vi "Configure Trip Line.vi"(0 "VISA resource name":refnum<visa-resource-name>, 1 "Display Position (50)":i32=50 max=100 step=1, 2 "Color":cluster{"R":i32, "G":i32, "B":i32} {"B" min=0 max=255 step=1; "G" min=0 max=255 step=1; "R" min=0 max=255 step=1}, 3 "Line Width (1: Normal)":i32(ring)=1 items=["Thin", "Normal", "Thick"], 5 "Group (1)":i32=1 min=1 max=60 step=1, 7 "Trip Line (1)":i32=1, 9 "Enable Trip Line (False)":bool, 11 "error in (no error)":errorcluster) -> (4 "VISA resource name out":refnum<visa-resource-name>, 6 "Group":i32, 8 "Trip Line":i32, 15 "error out":errorcluster)   [LabVIEW 2020, in "Yokogawa GX Series.lvlib"]
doc: "Sets the trip line for a display group.\n\nCommand: STripLine"
uses:
  <instrlib>/Yokogawa GX Series/Yokogawa GX Series.lvlib
panel:
  # "%"
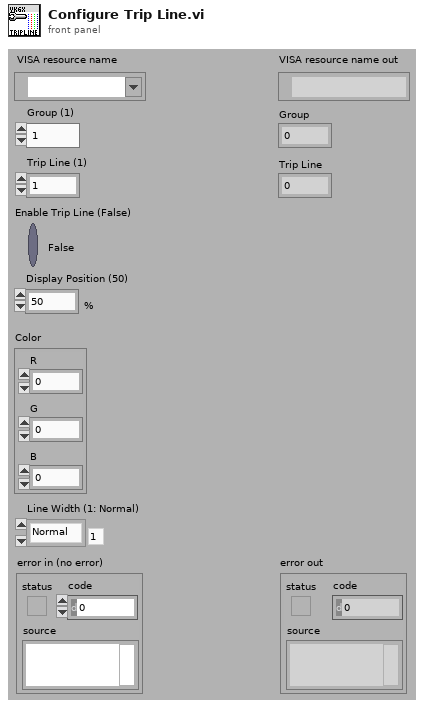
[diagram p1: front panel]
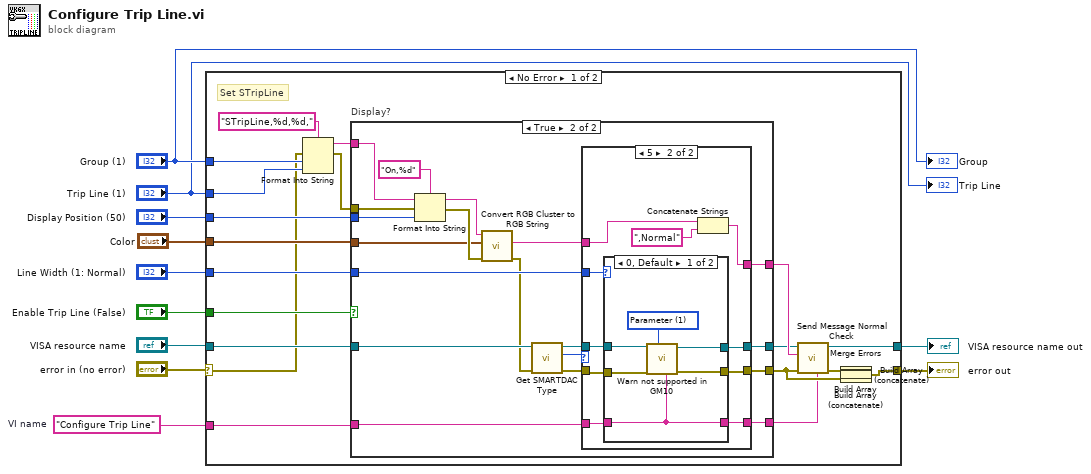
[diagram p0: block diagram]
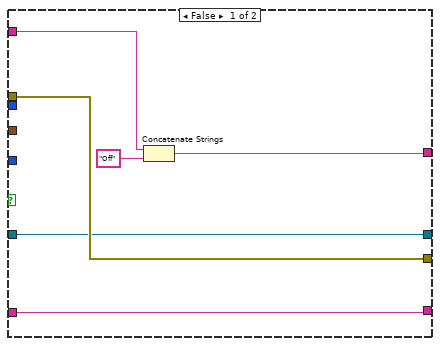
[diagram p2: hidden frame]
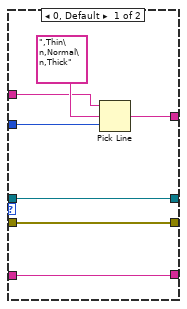
[diagram p3: hidden frame]
diagram:
  w9 = "Configure Trip Line"  # VI name
  n1 = case shown="No Error" "error in (no error)" {
    selector: "error in (no error)" -> [w15 w85]
    tunnel: "Enable Trip Line (False)" -> [w33 _]
    tunnel: "Display Position (50)" -> [w32 _]
    tunnel: w9 -> [w21 _]
    tunnel: "Line Width (1: Normal)" -> [w30 _]
    tunnel: [w29 w86] -> w7
    tunnel: [w19 w85] -> w6
    tunnel: "Color" -> [w25 _]
    tunnel: "VISA resource name" -> [w16 w86]
    tunnel: "Group (1)" -> [w24 _]
    tunnel: "Trip Line (1)" -> [w23 _]
    frame No Error {
      # "Set STripLine"
      n2 = Format Into String(format string="STripLine,%d,%d,", error in=w15, w24, w23) -> (resulting string=w26:string, error out=w27:errorcluster)  [unwired: 1 in]
      n3 = case "Display?" shown="True" w33 {
        tunnel: w27 -> [w39 w58]
        tunnel: [w39 w47] -> w18
        tunnel: w26 -> [w38 w56]
        tunnel: [w36 w52] -> w31
        tunnel: w32 -> [_ w57]
        tunnel: w30 -> [_ w53]
        tunnel: w25 -> [_ w54]
        tunnel: w16 -> [w35 w43]
        tunnel: [w35 w48] -> w22
        tunnel: w21 -> [w34 w46]
        tunnel: [w34 w45] -> w17
        frame False {
          n4 = Concatenate Strings(w38, "Off") -> (w36:string)
        }
        frame True {
          n5 = Format Into String(format string="On,%d", initial string=w56, error in=w58, w57) -> (resulting string=w49:string, error out=w55:errorcluster)
          n6 = call <instrlib>:"Convert RGB Cluster to RGB String.vi"("error in (no error)"=w55, "RGB"=w54, "Initial String"=w49) -> ("error out"=w42:errorcluster, "RGB String"=w50:string)  [unwired: 7 in]
          n7 = call <instrlib>:"Get SMARTDAC Type.vi"("error in (no error)"=w42, "VISA resource name"=w43) -> ("error out"=w41:errorcluster, "SMARTDAC+ Type"=w40:u16, "VISA resource name out"=w44:refnum<visa-resource-name>)  [unwired: 7 in]
          n8 = case shown="5" w40 {
            tunnel: w53 -> [w65 w75]
            tunnel: [w63 w70] -> w52
            tunnel: w50 -> [w62 w71]
            tunnel: w44 -> [w60 w74]
            tunnel: [w60 w68] -> w48
            tunnel: w41 -> [w61 w73]
            tunnel: [w61 w67] -> w47
            tunnel: w46 -> [w59 w69]
            tunnel: [w59 w66] -> w45
            frame 0, Default {
              n9 = Pick Line(string ("")=w62, multi-line string=",Thin\n,Normal\n,Thick", line index=w65) -> (output string=w63:string)
            }
            frame 5 {
              n10 = case shown="0, Default" w75 {
                tunnel: w74 -> [w81 w84]
                tunnel: w73 -> [w76 w83]
                tunnel: w69 -> [w77 w82]
                tunnel: [w79 w84] -> w68
                tunnel: [w78 w83] -> w67
                tunnel: [w77 w82] -> w66
                frame 0, Default {
                  w80 = u16 1 items=["Command", "Parameter"] ("Kind (0: Command)")
                  n11 = call <instrlib>:"Warn not supported in GM10.vi"("Source (\"\")"=w77, "Kind (0: Command)"=w80, "error in (no error)"=w76, "VISA resource name"=w81) -> ("error out"=w78:errorcluster, "VISA resource name out"=w79:refnum<visa-resource-name>)  [unwired: 6 in]
                }
                frame 1 {
                }
              }
              n12 = Concatenate Strings(w71, ",Normal") -> (w70:string)
            }
          }
        }
      }
      n13 = call <instrlib>:"Send Message Normal Check.vi"("Source (\"\")"=w17, "error in (no error)"=w18, "Send Message (\"\")"=w31, "VISA resource name"=w22) -> ("error out"=w20:errorcluster, "VISA resource name out"=w29:refnum<visa-resource-name>)  [unwired: 2 in, 4 out]
      n14 = Build Array(w20, w18) -> (w14:errorcluster[])
      n15 = Build Array (concatenate)(w14) -> (w13:errorcluster[])
      n16 = Build Array (concatenate)(w13) -> (w12:errorcluster[])
      n17 = Merge Errors(w12) -> (w19:errorcluster)
    }
    frame Error {
    }
  }
  "error out" <- w6
  "VISA resource name out" <- w7
  "Group" <- "Group (1)"
  "Trip Line" <- "Trip Line (1)"
